vi "Measurement Logic.vi"(8 "error in":errorcluster, 10 "measurement configuration":T3={"relay name"="SiteRelay1", "channel"="K0", "relay action"=21} {"relay action" items=["Open Relay"=20, "Close Relay"=21]}, 11 "measure call context in":refnum<class "Measure Call Context.lvclass">) -> (0 "error out":errorcluster, 2 "measurement results":T1={"initial relay position"=10, "final relay position"=10} {"final relay position" items=["Open"=10, "Closed"=11]; "initial relay position" items=["Open"=10, "Closed"=11]}, 3 "measure call context out":refnum<class "Measure Call Context.lvclass">)   [LabVIEW 2021, in "NISwitchControlRelay.lvlib"]
uses:
  NISwitchControlRelay.lvlib
  <vilib>/Plug-In SDKs/Measurements/Measure Call Context/Measure Call Context.lvclass
  Measurement Configuration.ctl
  <instrlib>/niSwitch/niSwitch.llb/niSwitch Relay Action.ctl
  Measurement Results.ctl
  <instrlib>/niSwitch/niSwitch.llb/niSwitch Relay Position.ctl
  <instrlib>/niSwitch/niSwitch.llb/niSwitch Topologies.ctl
  <vilib>/Plug-In SDKs/Measurements/Measure Call Context/Reserve Sessions - 1Pin.vi
  <vilib>/Plug-In SDKs/Sessions/niSwitch/Initialize Sessions - 1Sess.vi
  <vilib>/Plug-In SDKs/Clients/Session Management V1/Session Reservation/Session Reservation.lvclass
  <vilib>/Plug-In SDKs/Sessions/niSwitch/Session Management niSwitch.lvlib
  <vilib>/Plug-In SDKs/Sessions/niSwitch/Session Factory/Session Factory.lvclass
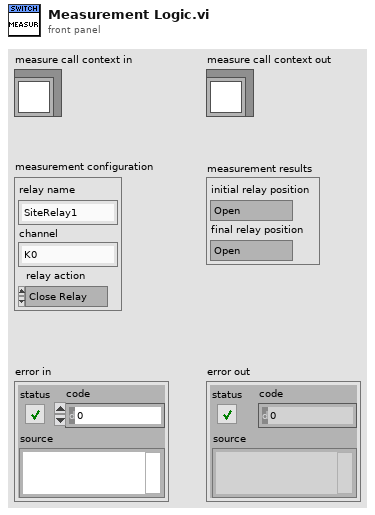
[diagram p1: front panel]
types:
  T1 = typedef "NISwitchControlRelay.lvlib/Measurement Results.ctl" = cluster{"initial relay position":T2, "final relay position":T2}
  T2 = typedef "niSwitch Relay Position.ctl" = i32
  T3 = typedef "NISwitchControlRelay.lvlib/Measurement Configuration.ctl" = cluster{"relay name":string, "channel":string, "relay action":T4}
  T4 = typedef "niSwitch Relay Action.ctl" = i32
  T5 = typedef "niSwitch Topologies.ctl" = string
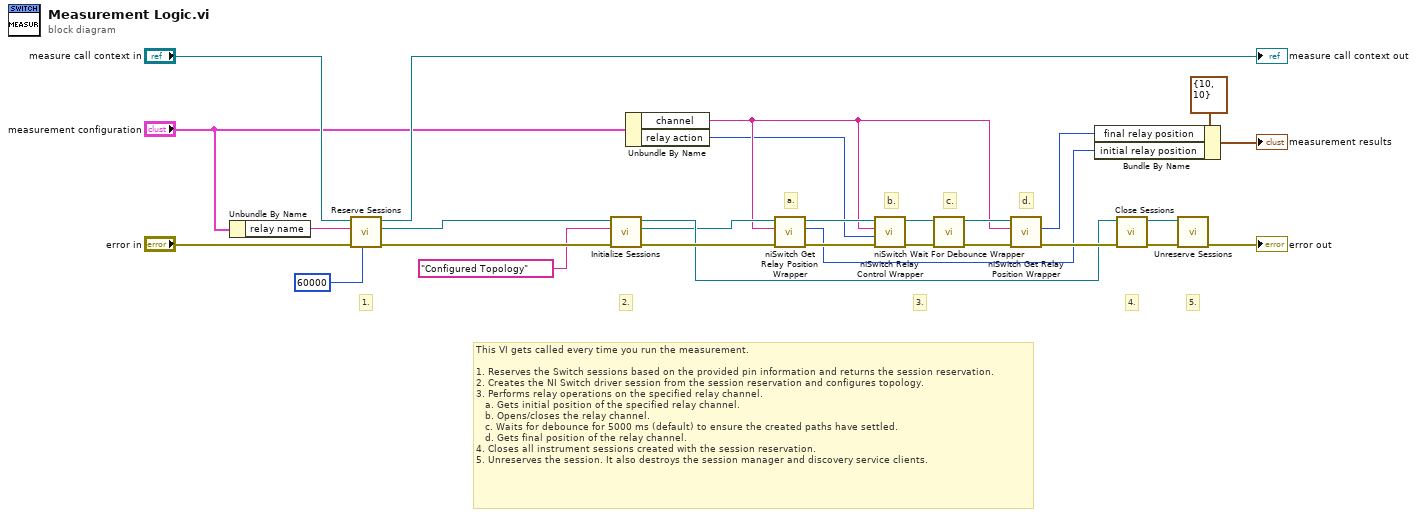
[diagram p0: block diagram]
diagram:
  # "d."
  # "c."
  # "b."
  # "a."
  # "5."
  # "4."
  # "3."
  # "2."
  # "1."
  # "This VI gets called every time you run the measurement.\n\n1. Reserves the Switch sessions based on the provided pin information and returns the session reservation.\n2. Creates the NI Switch driver session from the session reservation and configures topology. \n3. Performs relay operations on the specified relay channel.\n   a. Gets initial position of the specified relay channel.\n   b. Opens/closes the relay channel.\n   c. Waits for debounce for 5000 ms (default) to ensure the created paths have settled.\n   d. Gets final position of the relay channel.\n4. Closes all instrument sessions created with the session reservation.\n5. Unreserves the session. It also destroys the session manager and discovery service clients."
  n1 = Unbundle By Name("measurement configuration") -> ("relay name"=w8:string)
  n2 = call-poly <vilib>:"Reserve Sessions.vi"("timeout (ms)"=60000, "error in"="error in", "pin or relay name"=w8, "measurement context in"="measure call context in") -> ("error out"=w28:errorcluster, "session reservation out"=w27:refnum<class "Session Reservation.lvclass">, "measurement context out"=→"measure call context out":refnum<class "Measure Call Context.lvclass">)  [unwired: 5 in]
  n3 = call-poly <vilib>:"Initialize Sessions.vi"("error in"=w28, "topology name"=T5 "Configured Topology", "session reservation in"=w27) -> ("error out"=w15:errorcluster, "session"=w11:refnum<class "Session Factory.lvclass">, "session reservation out"=w12:refnum<class "Session Reservation.lvclass">)  [unwired: 5 in, 1 out]
  n4 = Unbundle By Name("measurement configuration") -> ("channel"=w10:string, "relay action"=w1:T4)
  n5 = call <vilib>:"niSwitch Get Relay Position Wrapper.vi"("error in"=w15, "relay name"=w10, "session factory in"=w11) -> ("error out"=w19:errorcluster, "position"=w13:T2, "session factory out"=w22:refnum<class "Session Factory.lvclass">)  [unwired: 6 in]
  n6 = call <vilib>:"niSwitch Relay Control Wrapper.vi"("error in"=w19, "relay action (Close Relay)"=w1, "relay names"=w10, "session factory in"=w22) -> ("error out"=w18:errorcluster, "session factory out"=w21:refnum<class "Session Factory.lvclass">)  [unwired: 6 in]
  n7 = call <vilib>:"niSwitch Wait For Debounce Wrapper.vi"("error in"=w18, "session factory in"=w21) -> ("error out"=w17:errorcluster, "session factory out"=w20:refnum<class "Session Factory.lvclass">)  [unwired: 8 in]
  n8 = call <vilib>:"niSwitch Get Relay Position Wrapper.vi"("error in"=w17, "relay name"=w10, "session factory in"=w20) -> ("error out"=w14:errorcluster, "position"=w16:T2)  [unwired: 6 in, 1 out]
  n9 = Bundle By Name(cluster=T1 {"initial relay position"=10, "final relay position"=10} ("measurement results"), "final relay position"=w16, "initial relay position"=w13) -> (→"measurement results":T1)
  n10 = call <vilib>:"Close Sessions.vi"("error in"=w14, "session reservation in"=w12) -> ("error out"=w25:errorcluster, "session reservation out"=w26:refnum<class "Session Reservation.lvclass">)  [unwired: 8 in]
  n11 = call <vilib>:"Unreserve Sessions.vi"("error in"=w25, "session reservation in"=w26) -> ("error out"=→"error out":errorcluster)  [unwired: 9 in]
